vi "LVClass_CameraSet ReadFile CameraParametersSetup.vi"(0 "CameraSet in":refnum<class "CameraSet.lvclass">, 11 "error in (no error)":errorcluster) -> (4 "CameraSet out":refnum<class "CameraSet.lvclass">, 15 "error out":errorcluster)   [LabVIEW 2020, in "CameraSet.lvclass"]
uses:
  CameraSet.lvclass
  CameraSet.lvclass/CameraSet.ctl
  CameraParametersSetup.ctl
  CameraParameters_Type.ctl
  <userlib>/_OpenG.lib/file/file.llb/File Exists - Scalar__ogtk.vi
  Read From XML File(array).vi
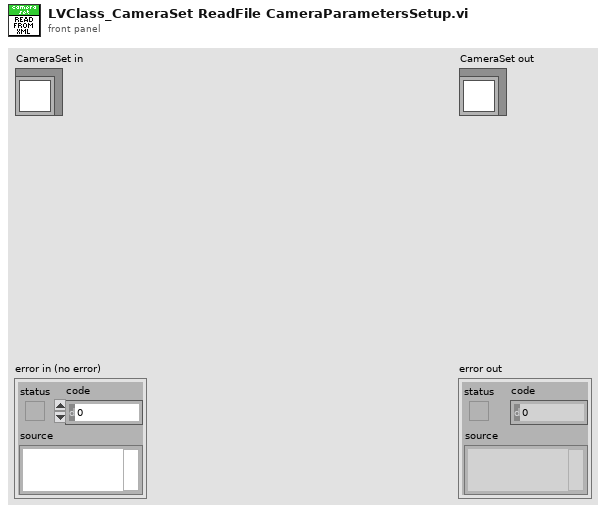
[diagram p1: front panel]
types:
  T1 = typedef "CameraParametersSetup.ctl" = cluster{"Name":string, "Type":T2, "Value":dbl, "BooleanValue":bool, "StringValue":string, "ConnectionParameter":bool}
  T2 = typedef "CameraParameters_Type.ctl" = enum16{"Integer", "Real", "String", "Boolean"}
  T3 = typedef "ParameterID.ctl" = cluster{"Name":string, "ConnectionParameter?":bool, "Type":T2, "Authorization":T4, "OnFlyAuthorization":T5, "StringValue":string, "Value":dbl, "Min":dbl, "Max":dbl, "BooleanValue":bool, "StringParameterList":string[]}
  T4 = typedef "CameraParameters_Authorization.ctl" = enum16{"Disable", "Gettable", "Settable - Gettable"}
  T5 = typedef "CameraParameters_OnFlyAuthorization.ctl" = enum16{"None", "Gettable", "Settable", "Settable - Gettable"}
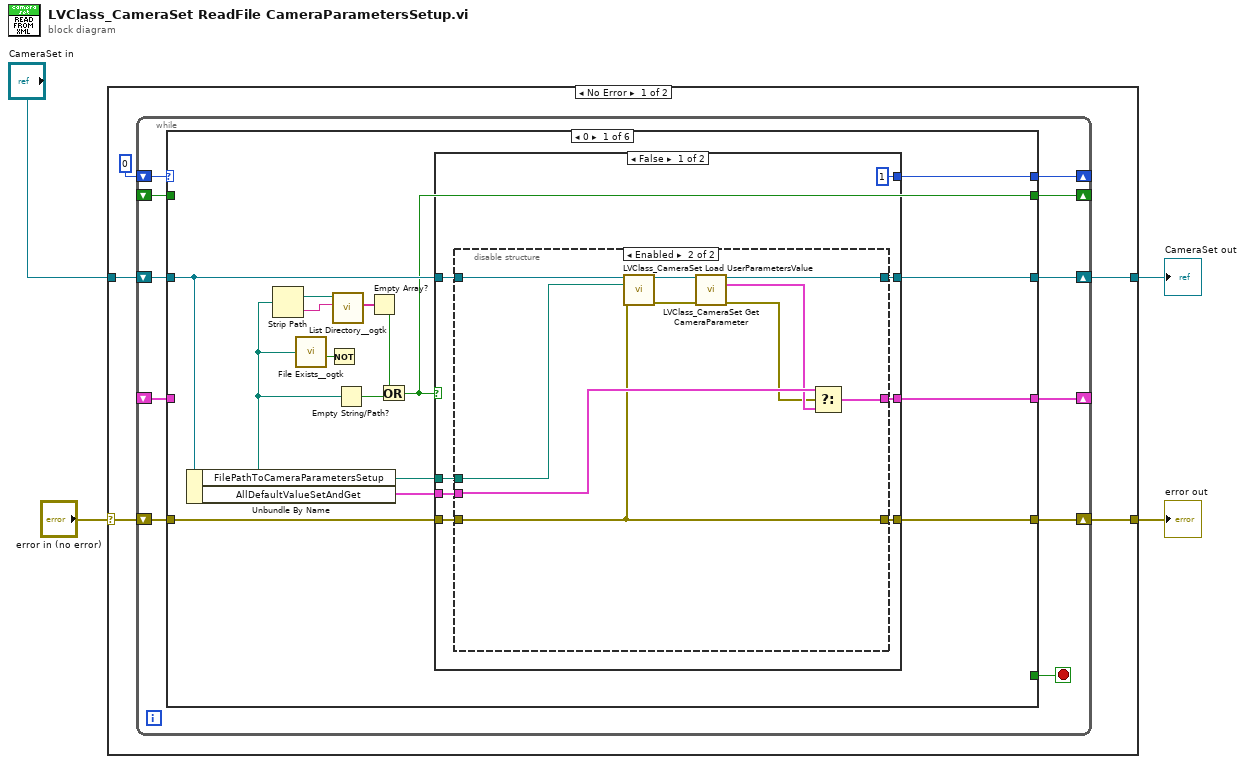
[diagram p0: block diagram]
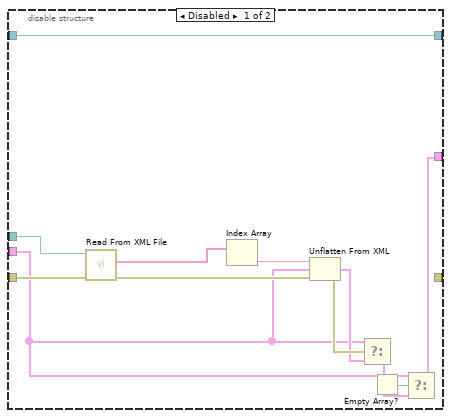
[diagram p2: hidden frame]
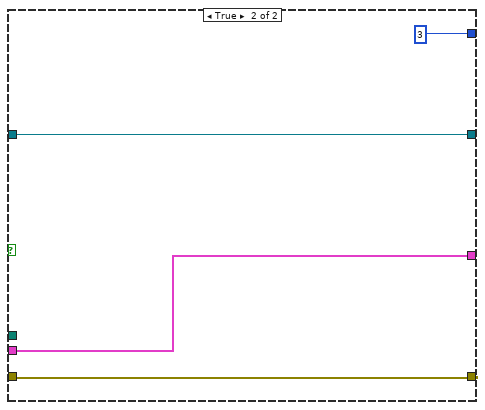
[diagram p3: hidden frame]
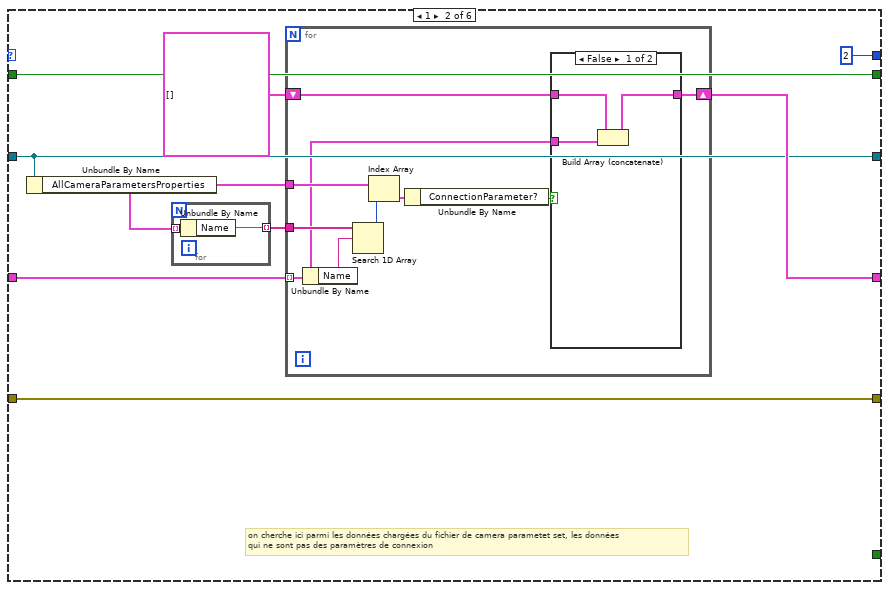
[diagram p4: hidden frame]
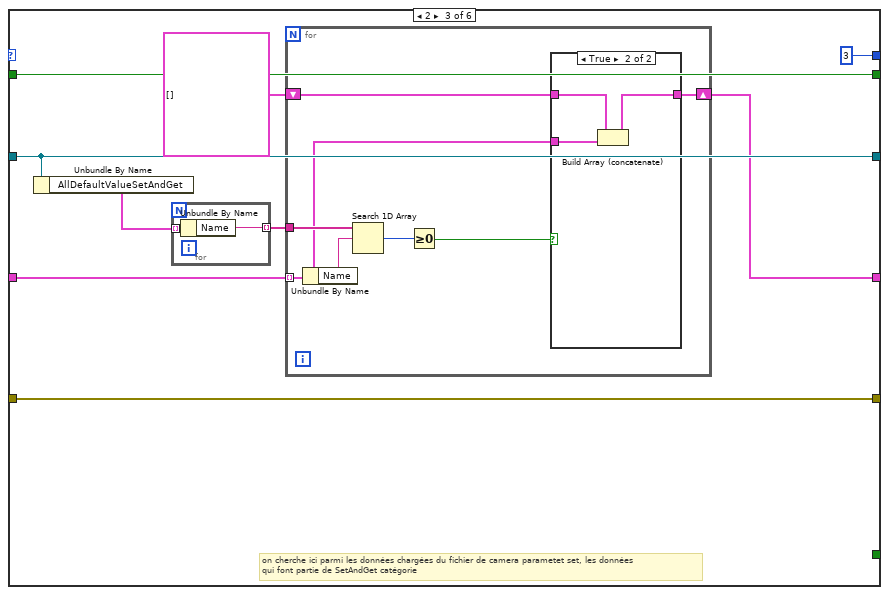
[diagram p6: hidden frame]
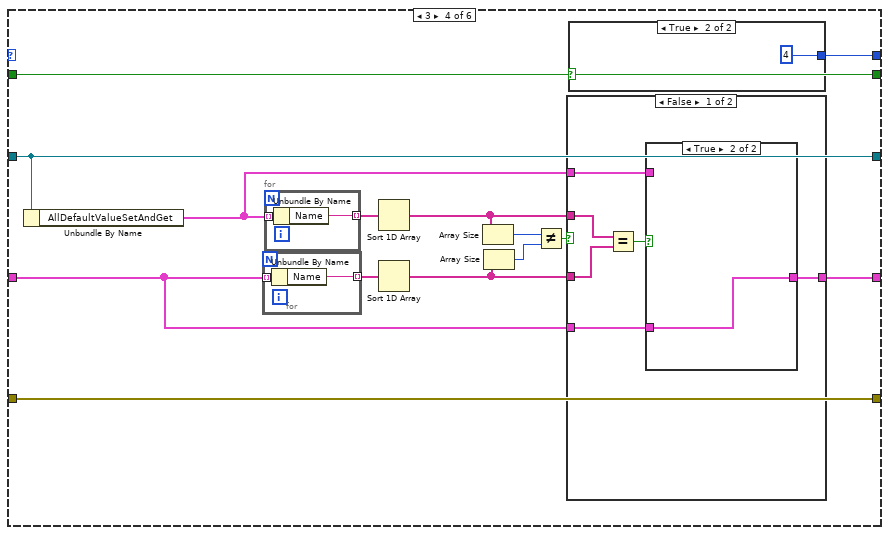
[diagram p8: hidden frame]
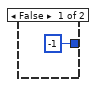
[diagram p9: hidden frame]
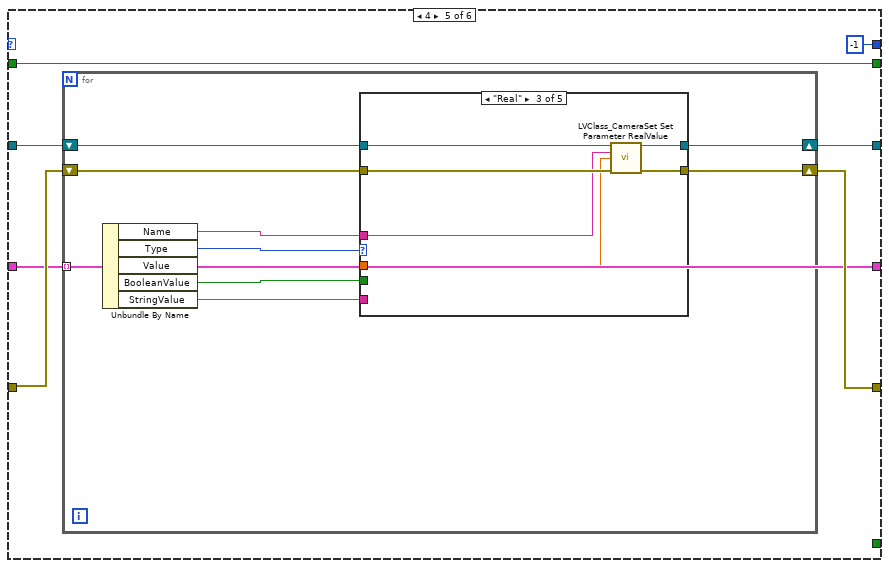
[diagram p12: hidden frame]
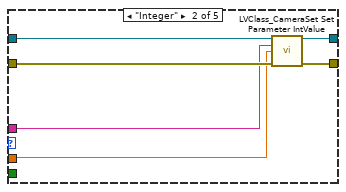
[diagram p14: hidden frame]
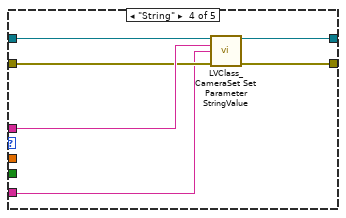
[diagram p15: hidden frame]
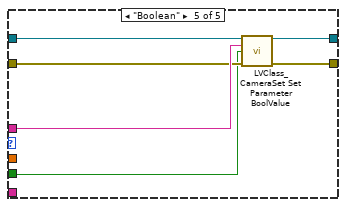
[diagram p16: hidden frame]
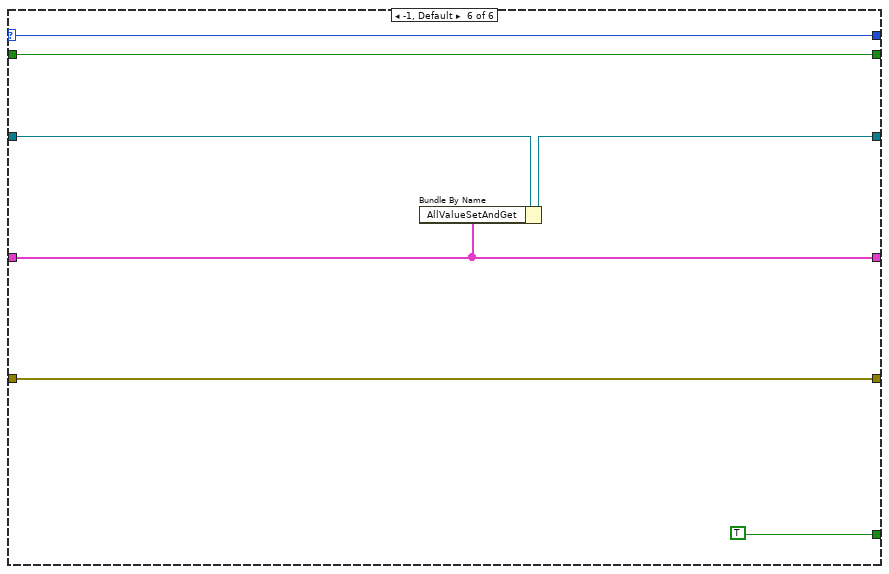
[diagram p17: hidden frame]
diagram:
  n1 = case shown="No Error" "error in (no error)" {
    selector: "error in (no error)" -> [w8 w196]
    tunnel: [w9 w196] -> w3
    tunnel: "CameraSet in" -> [w6 w195]
    tunnel: [w5 w195] -> w1
    frame No Error {
      n2 = while {
        shift-right: [w18] -> _
        shift-left: _ -> [w14]
        shift-right: [w12] -> _
        shift-left: 0 -> [w16]
        shift-right: [w13] -> w5
        shift-left: w6 -> [w17]
        shift-right: [w20] -> w9
        shift-left: w8 -> [w19]
        shift-right: [w11] -> _
        shift-left: _ -> [w10]
        stop <- w15 stop-if-true
        n3 = case shown="0" w16 {
          selector: w16 -> [_ _ _ _ _ w192]
          tunnel: [w35 w77 w101 w121 w147 w193] -> w20
          tunnel: w19 -> [w34 w77 w101 w121 w148 w193]
          tunnel: [w33 w72 w95 w125 w146 w191] -> w18
          tunnel: w17 -> [w30 w71 w96 w129 w150 w190]
          tunnel: [_ _ _ _ _ TRUE] -> w15
          tunnel: w14 -> [_ w73 w97 w122 w146 w191]
          tunnel: [w29 w71 w96 w129 w149 w189] -> w13
          tunnel: [w31 2 3 w117 -1 w192] -> w12
          tunnel: [w21 w70 w94 w116 w145 w188] -> w11
          tunnel: w10 -> [_ w70 w94 w116 w145 w188]
          frame 0 {
            n4 = Unbundle By Name(w30) -> ("FilePathToCameraParametersSetup"=w23:path, "AllDefaultValueSetAndGet"=w32:T1[])
            n5 = Strip Path(path=w23) -> (stripped path=w26:path, name=w27:string)
            n6 = call-poly <userlib>:"File Exists__ogtk.vi"("file path"=w23) -> ("exists"=w28:bool)  [unwired: 6 in, 1 out]
            n7 = Not(x=w28) -> ()  [unwired: 1 out]
            n8 = call <userlib>:"List Directory__ogtk.vi"("pattern"=w27, "directory path"=w26) -> ("file names"=w25:string[])  [unwired: 2 in, 3 out]
            n9 = Empty String/Path?(string/path=w23) -> (empty?=w22:bool)
            n10 = Empty Array?(array=w25) -> (empty?=w24:bool)
            n11 = Or(x=w24, y=w22) -> (x .or. y?=w21:bool)
            n12 = case shown="False" w21 {
              tunnel: w23 -> [w43 _]
              tunnel: [w36 w69] -> w35
              tunnel: w34 -> [w42 w69]
              tunnel: [w41 w68] -> w33
              tunnel: w32 -> [w40 w68]
              tunnel: [1 3] -> w31
              tunnel: w30 -> [w38 w66]
              tunnel: [w37 w66] -> w29
              frame False {
                n13 = disable-structure shown="Enabled" {
                  disable-tunnel: w43 -> [w52 w64]
                  disable-tunnel: w42 -> [w51 w57]
                  disable-tunnel: [w46 w62] -> w41
                  disable-tunnel: w40 -> [w45 w63]
                  disable-tunnel: w38 -> [w44 w65]
                  disable-tunnel: [w44 w60] -> w37
                  disable-tunnel: [_ w57] -> w36
                  frame Disabled {
                    n14 = call-poly "Read From XML File.vi"("error in (no error)"=w51, "XML File Path"=w52) -> ("error out"=w55:errorcluster, "XML Elements"=w54:string[])  [unwired: 7 in, 1 out]
                    n15 = Index Array(array=w54) -> (element=w53:string)  [unwired: 1 in]
                    n16 = Unflatten From XML(xml string=w53, type=w45, error in (no error)=w55) -> (value=w49:T1[], error out=w50:errorcluster)
                    n17 = Select(t=w45, s=w50, f=w49) -> (s? t:f=w47:T1[])
                    n18 = Empty Array?(array=w47) -> (empty?=w48:bool)
                    n19 = Select(t=w45, s=w48, f=w47) -> (s? t:f=w46:T1[])
                  }
                  frame Enabled {
                    n20 = call "LVClass_CameraSet Load UserParametersValue.vi"("CameraSet.lvclass"=w65, "ParametersValue file path"=w64, "error in (no error)"=w57) -> ("CameraSet.lvclass"=w61:refnum<class "CameraSet.lvclass">, "error out"=w59:errorcluster)  [unwired: 11 in]
                    n21 = call "LVClass_CameraSet Get CameraParameter.vi"("CameraSet in"=w61, "error in (no error)"=w59) -> ("CameraSet out"=w60:refnum<class "CameraSet.lvclass">, "AllCurrentValueSetAndGet"=w58:T1[], "error out"=w56:errorcluster)  [unwired: 10 in, 1 out]
                    n22 = Select(t=w63, s=w56, f=w58) -> (s? t:f=w62:T1[])
                  }
                }
              }
              frame True {
              }
            }
          }
          frame 1 {
            # "on cherche ici parmi les données chargées du fichier de camera parametet set, les données \nqui ne sont pas des paramètres de connexion"
            n23 = Unbundle By Name(w71) -> ("AllCameraParametersProperties"=w75:T3[])
            n24 = for {
              tunnel: w75 -> [w80] mode=indexing
              tunnel: [w79] -> w76 mode=indexing
              n25 = Unbundle By Name(w80) -> ("Name"=w79:string)
            }
            n26 = for {
              tunnel: w76 -> [w89]
              tunnel: w73 -> [w83] mode=indexing
              tunnel: w75 -> [w87]
              shift-right: [w84] -> w72
              shift-left: T1[] [] -> [w85]
              n27 = Unbundle By Name(w83) -> ("Name"=w88:string)
              n28 = Search 1D Array(1D array=w89, element=w88) -> (index of element=w86:i32)  [unwired: 1 in]
              n29 = Index Array(array=w87, index=w86) -> (element=w82:T3)
              n30 = Unbundle By Name(w82) -> ("ConnectionParameter?"=w81:bool)
              n31 = case shown="False" w81 {
                tunnel: w85 -> [w92 w93]
                tunnel: [w91 w93] -> w84
                tunnel: w83 -> [w90 _]
                frame False {
                  n32 = Build Array (concatenate)(w92, w90) -> (w91:T1[])
                }
                frame True {
                }
              }
            }
          }
          frame 2 {
            # "on cherche ici parmi les données chargées du fichier de camera parametet set, les données \nqui font partie de SetAndGet catégorie"
            n33 = Unbundle By Name(w96) -> ("AllDefaultValueSetAndGet"=w99:T1[])
            n34 = for {
              tunnel: w99 -> [w104] mode=indexing
              tunnel: [w103] -> w100 mode=indexing
              n35 = Unbundle By Name(w104) -> ("Name"=w103:string)
            }
            n36 = for {
              tunnel: w100 -> [w111]
              tunnel: w97 -> [w107] mode=indexing
              shift-right: [w108] -> w95
              shift-left: T1[] [] -> [w109]
              n37 = Unbundle By Name(w107) -> ("Name"=w110:string)
              n38 = Search 1D Array(1D array=w111, element=w110) -> (index of element=w106:i32)  [unwired: 1 in]
              n39 = Greater Or Equal To 0?(x=w106) -> (x >= 0?=w105:bool)
              n40 = case shown="True" w105 {
                tunnel: w109 -> [w112 w115]
                tunnel: [w112 w114] -> w108
                tunnel: w107 -> [_ w113]
                frame False {
                }
                frame True {
                  n41 = Build Array (concatenate)(w115, w113) -> (w114:T1[])
                }
              }
            }
          }
          frame 3 {
            n42 = Unbundle By Name(w129) -> ("AllDefaultValueSetAndGet"=w118:T1[])
            n43 = for {
              tunnel: w122 -> [w144] mode=indexing
              tunnel: [w143] -> w123 mode=indexing
              n44 = Unbundle By Name(w144) -> ("Name"=w143:string)
            }
            n45 = for {
              tunnel: w118 -> [w142] mode=indexing
              tunnel: [w141] -> w124 mode=indexing
              n46 = Unbundle By Name(w142) -> ("Name"=w141:string)
            }
            n47 = Sort 1D Array(array=w124) -> (sorted array=w120:string[])
            n48 = Sort 1D Array(array=w123) -> (sorted array=w119:string[])
            n49 = Array Size(array=w120) -> (size(s)=w128:i32)
            n50 = Array Size(array=w119) -> (size(s)=w127:i32)
            n51 = Not Equal?(x=w128, y=w127) -> (x != y?=w126:bool)
            n52 = case shown="False" w126 {
              tunnel: w118 -> [w132 w140]
              tunnel: [w134 w140] -> w125
              tunnel: w120 -> [w137 _]
              tunnel: w119 -> [w136 _]
              tunnel: w122 -> [w133 _]
              frame False {
                n53 = Equal?(x=w137, y=w136) -> (x = y?=w135:bool)
                n54 = case shown="True" w135 {
                  tunnel: [w138 w139] -> w134
                  tunnel: w133 -> [_ w139]
                  tunnel: w132 -> [w138 _]
                  frame False {
                  }
                  frame True {
                  }
                }
              }
              frame True {
              }
            }
            n55 = case shown="True" w116 {
              tunnel: [-1 4] -> w117
              frame False {
              }
              frame True {
              }
            }
          }
          frame 4 {
            n56 = for {
              tunnel: w146 -> [w154] mode=indexing
              shift-right: [w155] -> w149
              shift-left: w150 -> [w156]
              shift-right: [w152] -> w147
              shift-left: w148 -> [w153]
              n57 = Unbundle By Name(w154) -> ("Name"=w157:string, "Type"=w161:T2, "Value"=w158:dbl, "BooleanValue"=w160:bool, "StringValue"=w159:string)
              n58 = case shown="\"Real\"" w161 {
                tunnel: w157 -> [_ w164 w171 w180 w186]
                tunnel: w156 -> [w163 w169 w175 w181 w187]
                tunnel: [w163 w167 w173 w178 w184] -> w155
                tunnel: [w162 w166 w172 w177 w183] -> w152
                tunnel: w153 -> [w162 w168 w174 w179 w185]
                tunnel: w158 -> [_ w165 w170 _ _]
                tunnel: w160 -> [_ _ _ _ w182]
                tunnel: w159 -> [_ _ _ w176 _]
                frame Default {
                }
                frame "Integer" {
                  n59 = call "LVClass_CameraSet Set Parameter IntValue.vi"("CameraSet.lvclass"=w169, "parameter_name"=w164, "Value"=w165, "error in (no error)"=w168) -> ("CameraSet.lvclass"=w167:refnum<class "CameraSet.lvclass">, "error out"=w166:errorcluster)  [unwired: 10 in]
                }
                frame "Real" {
                  n60 = call "LVClass_CameraSet Set Parameter RealValue.vi"("CameraSet.lvclass"=w175, "parameter_name"=w171, "Value"=w170, "error in (no error)"=w174) -> ("CameraSet.lvclass"=w173:refnum<class "CameraSet.lvclass">, "error out"=w172:errorcluster)  [unwired: 10 in]
                }
                frame "String" {
                  n61 = call "LVClass_CameraSet Set Parameter StringValue.vi"("CameraSet.lvclass"=w181, "parameter name"=w180, "Value"=w176, "error in (no error)"=w179) -> ("CameraSet.lvclass"=w178:refnum<class "CameraSet.lvclass">, "error out"=w177:errorcluster)  [unwired: 10 in]
                }
                frame "Boolean" {
                  n62 = call "LVClass_CameraSet Set Parameter BoolValue.vi"("CameraSet.lvclass"=w187, "parameter_name"=w186, "Value"=w182, "error in (no error)"=w185) -> ("CameraSet.lvclass"=w184:refnum<class "CameraSet.lvclass">, "error out"=w183:errorcluster)  [unwired: 10 in]
                }
              }
            }
          }
          frame -1, Default {
            n63 = Bundle By Name(cluster=w190, "AllValueSetAndGet"=w191) -> (w189:refnum<class "CameraSet.lvclass">)
          }
        }
      }
    }
    frame Error {
    }
  }
  "error out" <- w3
  "CameraSet out" <- w1
